vi "subLoggingReturnTrueConditionString.vi"(9 "True string":string, 10 "Initial string":string, 11 "Condition (T)":bool=TRUE) -> (3 "Log string":string)   [LabVIEW 2019, in "SolutionBuilder.lvlib" / "SolutionBuilder.lvclass"]
uses:
  SolutionBuilder.lvclass
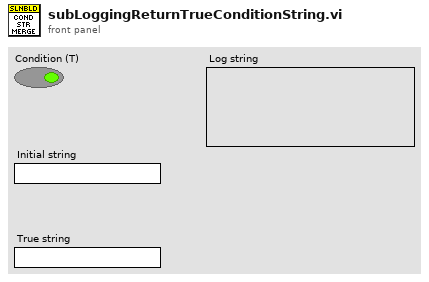
[diagram p1: front panel]
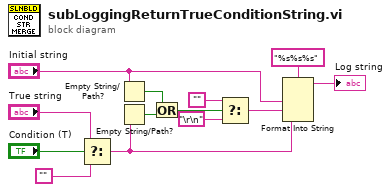
[diagram p0: block diagram]
diagram:
  n1 = Select(t="True string", s="Condition (T)", f="") -> (s? t:f=w3:string)
  n2 = Empty String/Path?(string/path="Initial string") -> (empty?=w9:bool)
  n3 = Empty String/Path?(string/path=w3) -> (empty?=w10:bool)
  n4 = Or(x=w9, y=w10) -> (x .or. y?=w8:bool)
  n5 = Select(t="", s=w8, f="\r\n") -> (s? t:f=w5:string)
  n6 = Format Into String(format string="%s%s%s", "Initial string", w5, w3) -> (resulting string=→"Log string":string)  [unwired: 2 in, 1 out]
